vi "get32bitIntegerArray.vi"() -> (3 "out32bi Integer Array":i32[](array[numeric]))   [LabVIEW 2014]
uses:
  GlobalVariables.vi
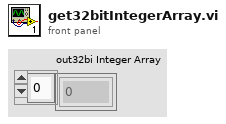
[diagram p1: front panel]
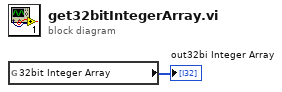
[diagram p0: block diagram]
diagram:
  n1 = global read "GlobalVariables.vi" "32bit Integer Array"() -> (→"out32bi Integer Array":i32[])
